vi "Save_Log.vi"(1 "Log File Path":path caption="selected path") -> ()   [LabVIEW 2011]
doc: "This VI saves the current global log text to a plaintext file of the user's choice."
uses:
  low_level_proc/globals.vi
panel:
  out "Error Out":errorcluster caption="error out"
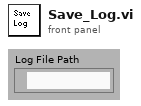
[diagram p1: front panel]
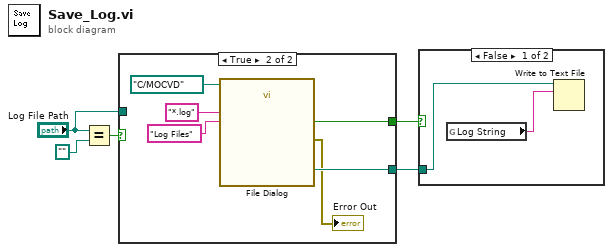
[diagram p0: block diagram]
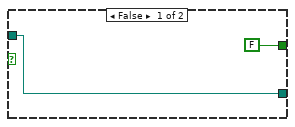
[diagram p2: hidden frame]
diagram:
  n1 = Equal?(x="Log File Path", y=path "") -> (x = y?=w2:bool)
  n2 = case shown="True" w2 {
    tunnel: [FALSE ("cancelled") w10] -> w5
    tunnel: [w7 w9] -> w4
    tunnel: "Log File Path" -> [w7 _]
    frame False {
    }
    frame True {
      n3 = call "File Dialog"("start path"=path "C:/MOCVD", "pattern (all files)"="*.log", "pattern label"="Log Files") -> ("selected path"=w9:path, "cancelled"=w10:bool, "error out"=→"Error Out":errorcluster)  [unwired: 4 in, 6 out]
    }
  }
  n4 = case shown="False" w5 {
    tunnel: w4 -> [w15 _]
    frame False {
      n5 = global read "globals.vi" "Log String"() -> (w14:string)
      n6 = Write to Text File(file (use dialog)=w15, text=w14) -> ()  [unwired: 1 in, 4 out]
    }
    frame True {
    }
  }
